vi "C4LV_readFeature.vi"   [LabVIEW 2015, in "libC4HdlLV.lvlib"]
uses:
  libC4HdlLV.lvlib
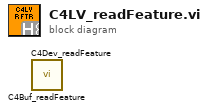
[diagram p0: block diagram]
diagram:
  n1 = call "C4Buf_readFeature.vi"() -> ()  [unwired: 13 in, 3 out]
  n2 = call "C4Dev_readFeature.vi"() -> ()  [unwired: 13 in, 3 out]
